vi "Format Mappings.vi"(4 "Destinations":string[](array[string]), 5 "Sources":string[](array[string])) -> (1 "Mappings":string[][](array[string]))   [LabVIEW 2016, in "System Mapping Tool.lvlib"]
uses:
  System Mapping Tool.lvlib
  <userlib>/_OpenG.lib/array/array.llb/Sort 1D Array (String)__ogtk.vi
  <userlib>/_OpenG.lib/array/array.llb/Reorder 2D Array2 (String)__ogtk.vi
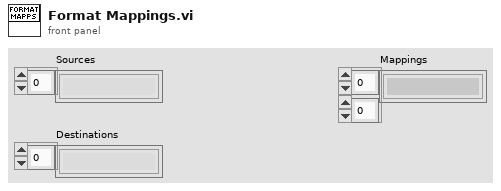
[diagram p1: front panel]
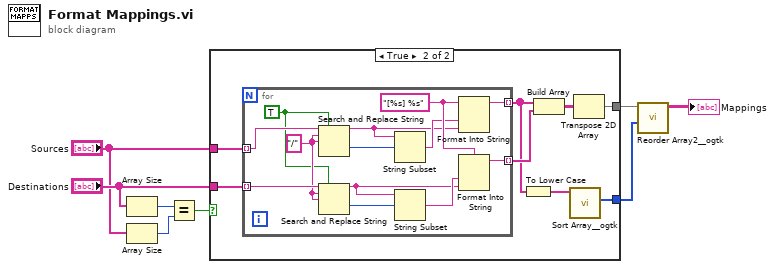
[diagram p0: block diagram]
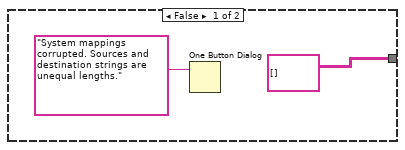
[diagram p2: hidden frame]
diagram:
  n1 = Array Size(array="Destinations") -> (size(s)=w8:i32)
  n2 = Array Size(array="Sources") -> (size(s)=w7:i32)
  n3 = Equal?(x=w8, y=w7) -> (x = y?=w6:bool)
  n4 = case shown="True" w6 {
    tunnel: [string[][] [] ("Mappings") w14] -> w3
    tunnel: "Destinations" -> [_ w17]
    tunnel: "Sources" -> [_ w18]
    tunnel: [_ w13] -> w1
    frame False {
      n5 = One Button Dialog(message="System mappings corrupted. Sources and destination strings are unequal lengths.") -> ()  [unwired: 1 in, 1 out]
    }
    frame True {
      n6 = for {
        tunnel: w18 -> [w31] mode=indexing
        tunnel: w17 -> [w30] mode=indexing
        tunnel: [w24] -> w11 mode=indexing
        tunnel: [w23] -> w16 mode=indexing
        w25 = "[%s] %s" ("format string")
        w28 = TRUE ("replace all? (F)")
        w29 = "/" ("search string")
        n7 = Search and Replace String(replace all?=w28, input string=w31, search string=w29, replace string=w29) -> (result string=w21:string, offset past replacement=w27:i32)  [unwired: 4 in, 2 out]
        n8 = Search and Replace String(replace all?=w28, input string=w30, search string=w29, replace string=w29) -> (result string=w19:string, offset past replacement=w26:i32)  [unwired: 4 in, 2 out]
        n9 = String Subset(string=w21, offset (0)=w27) -> (substring=w22:string)  [unwired: 1 in]
        n10 = String Subset(string=w19, offset (0)=w26) -> (substring=w20:string)  [unwired: 1 in]
        n11 = Format Into String(format string=w25, w22, w21) -> (resulting string=w24:string)  [unwired: 2 in, 1 out]
        n12 = Format Into String(format string=w25, w20, w19) -> (resulting string=w23:string)  [unwired: 2 in, 1 out]
      }
      n13 = To Lower Case(string=w11) -> (all lower case string=w12:string[])
      n14 = Build Array(w11, w16) -> (w15:string[][])
      n15 = call-poly <userlib>:"Sort Array__ogtk.vi"("Array in"=w12) -> ("Sorted Pointers"=w13:i32[])  [unwired: 9 in, 1 out]
      n16 = Transpose 2D Array(2D array=w15) -> (transposed array=w14:string[][])
    }
  }
  n17 = call-poly <userlib>:"Reorder Array2__ogtk.vi"("indices"=w1, "array"=w3) -> ("reordered array"=→"Mappings":string[][])  [unwired: 9 in]
